vi "Set ICP2-AO Changed Value.vi"(8 "error in (no error)":errorcluster, 9 "Value":dbl, 10 "AO Channel":T1, 11 "IO in":refnum<class "IO.lvclass">) -> (0 "error out":errorcluster, 3 "IO out":refnum<class "IO.lvclass">)   [LabVIEW 2022 SP3, in "IO.lvclass"]
uses:
  IO.lvclass
  Typedefs/ICP2-AO Channel Names.ctl
  Typedefs/API Command Cluster.ctl
  Typedefs/API Command Enum.ctl
  Typedefs/Device Names.ctl
  Typedefs/AO Value API Data.ctl
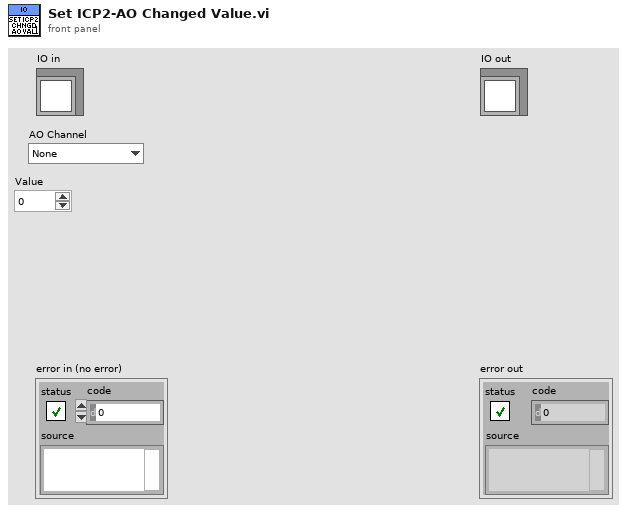
[diagram p1: front panel]
types:
  T1 = typedef "IO.lvclass/ICP2-AO Channel Names.ctl" = enum16{"None", "Recirc Pump Flow Set - R1", "Recirc Pump Flow Set - R2", "Recirc Pump Flow Set - R3", "Recirc Pump Flow Set - R4", "Recirc Pump Flow Set - R5", "Recirc Pump Flow Set - R6"}
  T2 = typedef "IO.lvclass/AO Value API Data.ctl" = cluster{"Device Name":T3, "Index":i32, "Value":dbl}
  T3 = typedef "IO.lvclass/Device Names.ctl" = enum16{"ICP1-DO", "ICP2-DI", "ICP2-DO", "ICP1-AI", "ICP1-AO", "ICP2-AO"}
  T4 = typedef "IO.lvclass/API Command Enum.ctl" = enum16{"Set DO Value", "Set AO Value", "Purge PH"}
  T5 = typedef "IO.lvclass/API Command Cluster.ctl" = cluster{"Command":T4, "Arguments":string, "Data":variant}
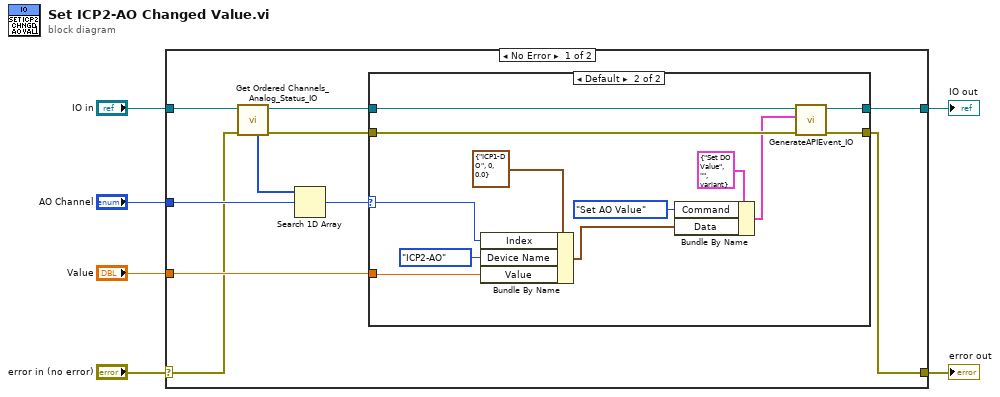
[diagram p0: block diagram]
diagram:
  n1 = case shown="No Error" "error in (no error)" {
    selector: "error in (no error)" -> [w10 w32]
    tunnel: [w9 w32] -> w5
    tunnel: [w13 w31] -> w3
    tunnel: "IO in" -> [w16 w31]
    tunnel: "AO Channel" -> [w15 _]
    tunnel: "Value" -> [w12 _]
    frame No Error {
      n2 = call-dynamic "Get Ordered Channels_Analog_Status_IO.vi"("error in (no error)"=w10, "IO in"=w16) -> ("error out"=w11:errorcluster, "IO out"=w14:refnum<class "IO.lvclass">, "Ordered ICP2-AO Channels"=w7:T1[])  [unwired: 5 in, 2 out]
      n3 = Search 1D Array(1D array=w7, element=w15) -> (index of element=w8:i32)  [unwired: 1 in]
      n4 = case shown="Default" w8 {
        selector: w8 -> [_ w23]
        tunnel: w14 -> [w18 w19]
        tunnel: [w18 w29] -> w13
        tunnel: w12 -> [_ w24]
        tunnel: w11 -> [w17 w30]
        tunnel: [w17 w28] -> w9
        frame -1 {
        }
        frame Default {
          n5 = Bundle By Name(cluster=T2 {"Device Name"=enum."ICP1-DO", "Index"=0, "Value"=0.0} ("DO Value Input"), "Index"=w23, "Device Name"=Device_Names."ICP2-AO", "Value"=w24) -> (w22:T2)
          n6 = Bundle By Name(cluster=T5 {"Command"=enum."Set DO Value", "Arguments"="", "Data"=variant} ("API Command Cluster"), "Command"=API_Command_Enum."Set AO Value", "Data"=w22) -> (w25:T5)
          n7 = call "GenerateAPIEvent_IO.vi"("error in (no error)"=w30, "API Command Cluster"=w25, "IO.lvclass"=w19) -> ("error out"=w28:errorcluster, "IO.lvclass out"=w29:refnum<class "IO.lvclass">)  [unwired: 7 in]
        }
      }
    }
    frame Error {
    }
  }
  "error out" <- w5
  "IO out" <- w3
